vi "saveGlobal.vi"() -> ()   [LabVIEW 2017, in "vi_tools.lvlib"]
doc: "<b>Changes</b> the defaults of all controls on the front panel to be the current values. <b>Saves the VI</b>."
uses:
  vi_tools.lvlib
  shared/shared.lvlib
panel:
  in  "message":string="Save Global must be launched from the Global Variable VI you wish to save."
  # "Wait while we process you Global Variable VI.\n\nChanges the defaults of all controls on the front panel to be the current values. Saves the VI."
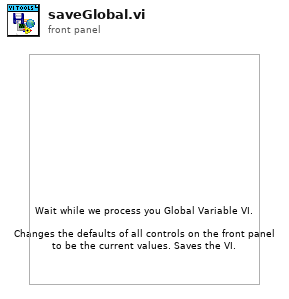
[diagram p1: front panel]
types:
  T1 = enum32{"Invalid", "Standard", "Closed", "Hidden", "Minimized", "Maximized"}
  T2 = enum32{"invalid VI type", "Standard VI", "Control VI", "Global VI", "Polymorphic VI", "Configuration VI", "SubSystem", "Facade VI", "Method VI", "Statechart Diagram VI"}
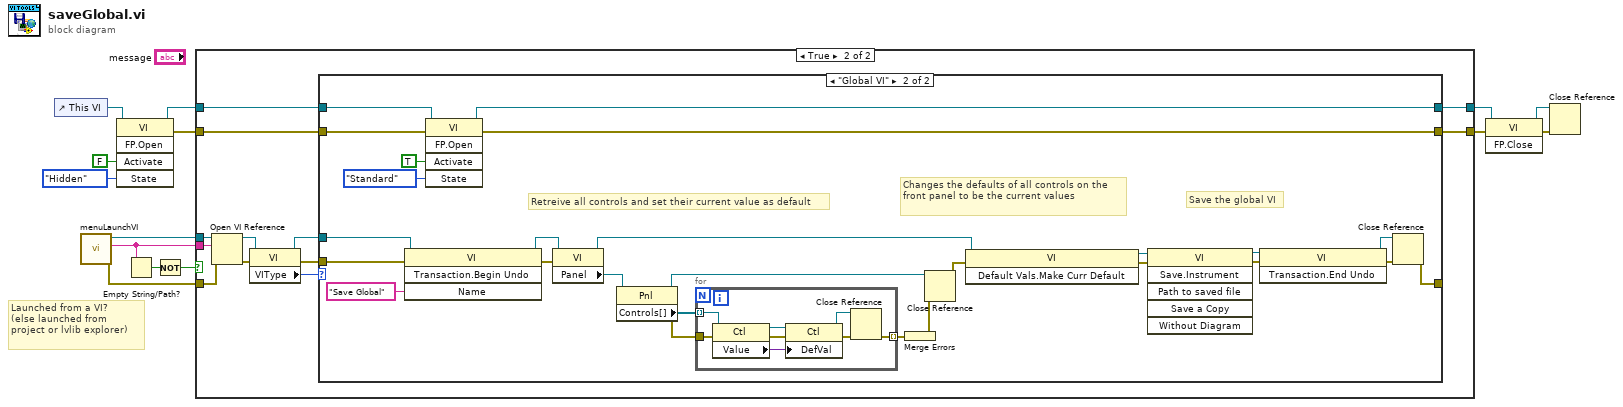
[diagram p0: block diagram]
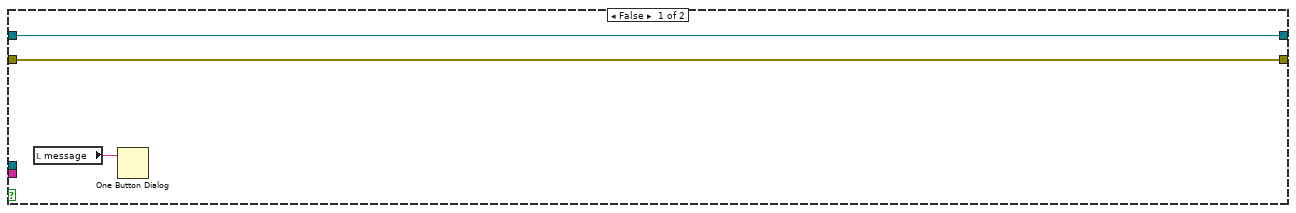
[diagram p2: hidden frame]
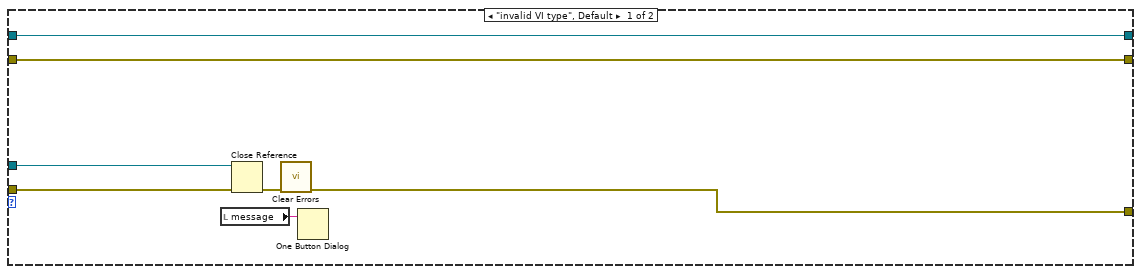
[diagram p3: hidden frame]
diagram:
  # "Launched from a VI?\n(else launched from project or lvlib explorer)"
  n1 = control-ref of="This VI"() -> (w4:refnum<vi>)
  n2 = call "menuLaunchVI.vi"() -> ("error out"=w1:errorcluster, "Menu Launch:VI"=w2:string, "Menu Launch:App"=w3:refnum<vi>)  [unwired: 9 in]
  n3 = invoke class="VI" method="FP.Open"(reference=w4, "Activate"=FALSE ("Activate?"), "State"=T1."Hidden") -> (reference out=w10:refnum<vi>, error out=w9:errorcluster)  [unwired: 2 in, 3 out]
  n4 = Empty String/Path?(string/path=w2) -> (empty?=w14:bool)
  n5 = Not(x=w14) -> (.not. x?=w13:bool)
  n6 = case shown="True" w13 {
    tunnel: w3 -> [_ w29]
    tunnel: w2 -> [_ w28]
    tunnel: w9 -> [w16 w20]
    tunnel: w10 -> [w15 w21]
    tunnel: [w16 w18] -> w11
    tunnel: [w15 w19] -> w12
    tunnel: w1 -> [_ w22]
    frame False {
      n7 = local read "message"() -> (w17:string)
      n8 = One Button Dialog(message=w17) -> ()  [unwired: 1 in, 1 out]
    }
    frame True {
      n9 = Open VI Reference(application reference (local)=w29, vi path=w28, error in (no error)=w22) -> (vi reference=w25:refnum<vi>, error out=w27:errorcluster)  [unwired: 3 in]
      n10 = property class="VI"(reference=w25, error in=w27) -> (reference out=w24:refnum<vi>, error out=w26:errorcluster, "VIType"=w23:T2)
      n11 = case shown="\"Global VI\"" w23 {
        tunnel: [w33 w62] -> _
        tunnel: w26 -> [w36 w51]
        tunnel: w24 -> [w35 w48]
        tunnel: w21 -> [w31 w40]
        tunnel: w20 -> [w30 w39]
        tunnel: [w31 w38] -> w19
        tunnel: [w30 w37] -> w18
        frame "invalid VI type", Default {
          n12 = local read "message"() -> (w32:string)
          n13 = Close Reference(reference=w35, error in (no error)=w36) -> (error out=w34:errorcluster)
          n14 = call <vilib>:"Clear Errors.vi"("error in (no error)"=w34) -> ("error out"=w33:errorcluster)  [unwired: 5 in, 1 out]
          n15 = One Button Dialog(message=w32) -> ()  [unwired: 1 in, 1 out]
        }
        frame "Global VI" {
          # "Save the global VI"
          # "Changes the defaults of all controls on the front panel to be the current values"
          # "Retreive all controls and set their current value as default"
          n16 = invoke class="VI" method="Transaction.Begin Undo"(reference=w48, error in=w51, "Name"="Save Global") -> (reference out=w49:refnum<vi>, error out=w50:errorcluster)  [unwired: 1 in, 2 out]
          n17 = invoke class="VI" method="FP.Open"(reference=w40, error in=w39, "Activate"=TRUE ("Activate?"), "State"=T1."Standard") -> (reference out=w38:refnum<vi>, error out=w37:errorcluster)  [unwired: 1 in, 3 out]
          n18 = property class="VI"(reference=w49, error in=w50) -> (reference out=w54:refnum<vi>, "Panel"=w61:refnum<vi>)  [unwired: 1 out]
          n19 = property class="Pnl"(reference=w61) -> (reference out=w58:refnum<vi>, error out=w59:errorcluster, "Controls[]"=w60:refnum<vi>[])  [unwired: 1 in]
          n20 = for {
            tunnel: w60 -> [w64] mode=indexing
            tunnel: [w67] -> w57 mode=indexing
            tunnel: w59 -> [w63]
            n21 = property class="Ctl"(reference=w64, error in=w63) -> (reference out=w70:refnum<vi>, error out=w68:errorcluster, "Value"=w69:variant)
            n22 = property class="Ctl"(reference=w70, error in=w68, "DefVal"=w69) -> (reference out=w65:refnum<vi>, error out=w66:errorcluster)
            n23 = Close Reference(reference=w65, error in (no error)=w66) -> (error out=w67:errorcluster)
          }
          n24 = Merge Errors(w57) -> (w56:errorcluster)
          n25 = Close Reference(reference=w58, error in (no error)=w56) -> (error out=w55:errorcluster)
          n26 = invoke class="VI" method="Default Vals.Make Curr Default"(reference=w54, error in=w55) -> (reference out=w53:refnum<vi>, error out=w52:errorcluster)  [unwired: 1 in, 1 out]
          n27 = invoke class="VI" method="Save.Instrument"(reference=w53, error in=w52) -> (reference out=w46:refnum<vi>, error out=w45:errorcluster)  [unwired: 4 in, 4 out]
          n28 = invoke class="VI" method="Transaction.End Undo"(reference=w46, error in=w45) -> (reference out=w43:refnum<vi>, error out=w44:errorcluster)  [unwired: 1 in, 1 out]
          n29 = Close Reference(reference=w43, error in (no error)=w44) -> (error out=w62:errorcluster)
        }
      }
    }
  }
  n30 = invoke class="VI" method="FP.Close"(reference=w12, error in=w11) -> (reference out=w5:refnum<vi>, error out=w6:errorcluster)  [unwired: 1 in, 1 out]
  n31 = Close Reference(reference=w5, error in (no error)=w6) -> ()  [unwired: 1 out]
